vi "Frame Page.vi"(8 "error in (no error)":errorcluster, 11 "Node Ptr":T2 format="%.0x") -> (0 "error out":errorcluster)   [LabVIEW 2019, in "Protection and Counter Addon System Explorer.lvlib"]
uses:
  Protection and Counter Addon System Explorer.lvlib
  <vilib>/NI VeriStand/Custom Device API/Custom Device Item Ref.ctl
  NationalInstruments.VeriStand.SystemStorageUI
  Types/Event Trigger Type.ctl
  <vilib>/NI VeriStand/UI Controls/Single Node Browser/Net Event Data.ctl
  <vilib>/NI VeriStand/UI Controls/Single Node Browser/Net Event.ctl
  Addon Shared/SubVIs/GUID Lookup.vi
  <vilib>/NI VeriStand/Custom Device API/Custom Device API.lvlib
  <vilib>/NI VeriStand/UI Controls/Single Node Browser/NI_VS UI Single Node Browser.lvlib
  Addon Shared/Protection and Counter Addon Shared.lvlib
panel:
  in  "Transmit Trigger":T1
  in  "Trigger":refnum<k24>(container)
  in  "Trigger Settings":cluster{"Section Name":string}={"Section Name"="Transmission Trigger"}
  in  "Trigger":refnum<k24>(container)
  in  "Disable Transmission":bool
  in  "Disable Settings":cluster{"Section Name":string}={"Section Name"="Disable Transmission"}
  in  "Description":string
  out "Frame ID":u32 format="%.0x"
  in  "Custom Device Settings":cluster{"Section Name":string}={"Section Name"="Frame Settings"}
  out "Name":string
  in  "SHDocVw.IWebBrowser2":refnum<k7>(container)
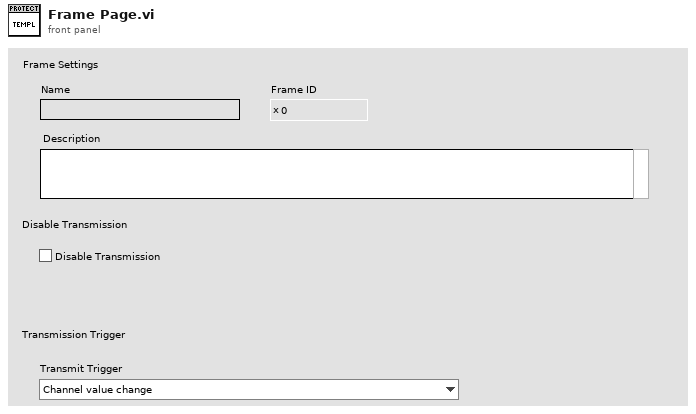
[diagram p1: front panel]
types:
  T1 = typedef "Protection and Counter Addon System Explorer.lvlib/Event Trigger Type.ctl" = enum16{"Channel value change", "Trigger channel (not zero)", "Channel value change or trigger channel (not zero)", "Trigger channel (any value change)", "Channel value change or trigger channel (any value change)"}
  T2 = typedef "Custom Device API.lvlib/Custom Device Item Ref.ctl" = u64
  T3 = cluster{"Trigger":refnum<user-event>, "Transmission":refnum<user-event>}
  T4 = typedef "Protection and Counter Addon System Explorer.lvlib/Frame Settings.ctl" = cluster{"ID":u32, "Disable Transmission":bool, "Disable Transmission Ref":T2, "Transmit Trigger":T1, "Transmit Trigger Ref":T2}
  T5 = typedef "Custom Device API.lvlib/Custom Device Item Info.ctl" = cluster{"Name":string, "Is Channel":bool, "GUID":string, "Is Waveform":bool}
  T6 = typedef "NI_VS UI Single Node Browser.lvlib/Single Node Browser Ref.ctl" = refnum<k24>
  T7 = typedef "NI_VS UI Single Node Browser.lvlib/Callback Type.ctl" = cluster{"Net Callbacks":refnum<k27>[], "Event":refnum<user-event>}
  T8 = typedef "Custom Device API.lvlib/Custom Device Commands.ctl" = enum16{"Default", "Item renamed", "Shutdown", "Dynamic button pressed"}
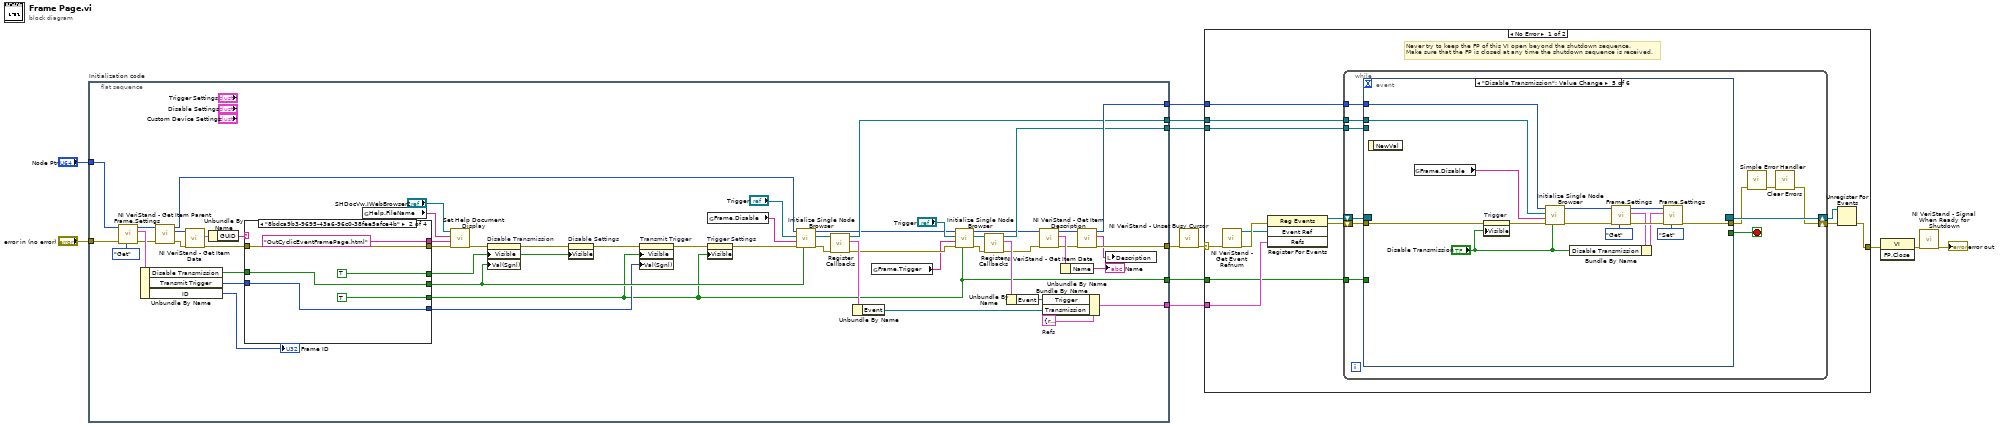
[diagram p0: block diagram]
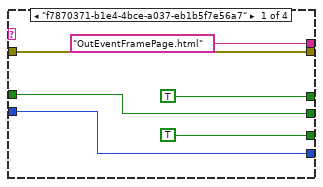
[diagram p2: hidden frame]
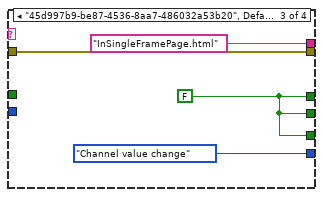
[diagram p3: hidden frame]
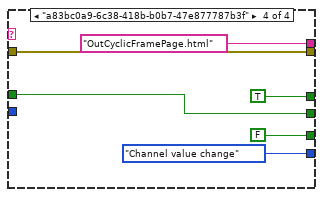
[diagram p4: hidden frame]
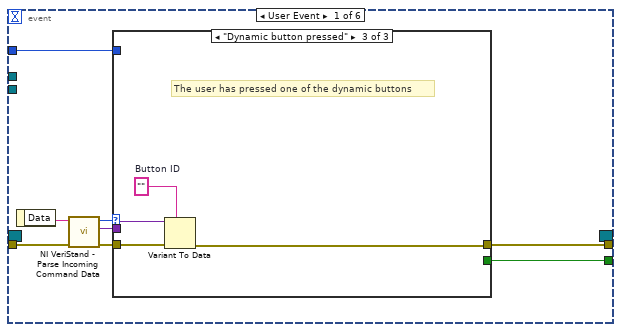
[diagram p5: hidden frame]
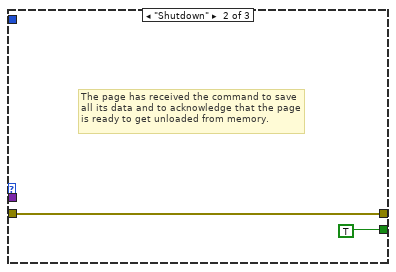
[diagram p7: hidden frame]
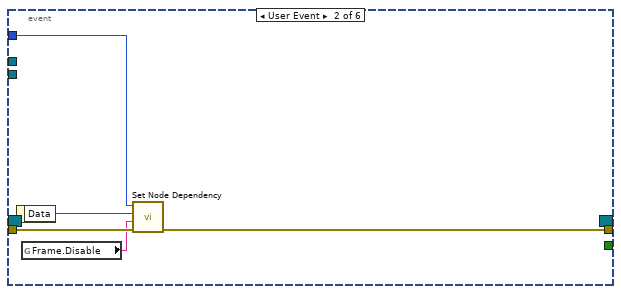
[diagram p8: hidden frame]
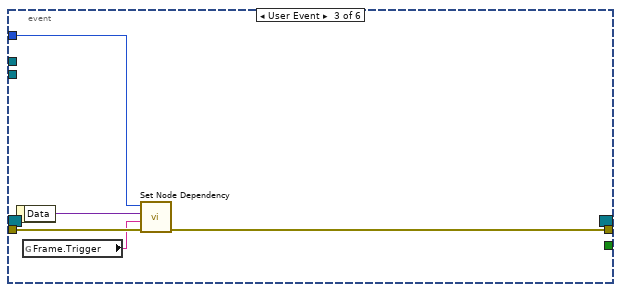
[diagram p9: hidden frame]
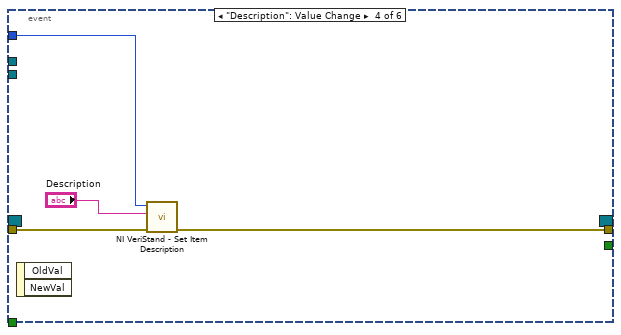
[diagram p10: hidden frame]
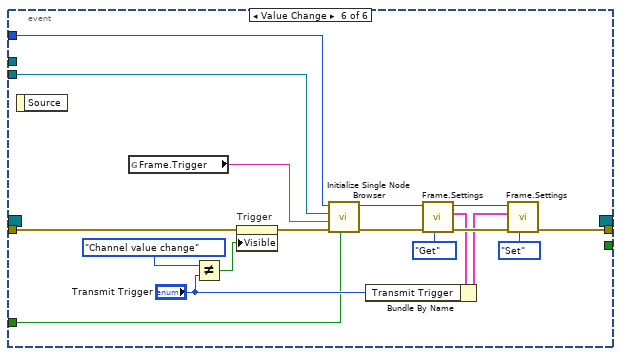
[diagram p11: hidden frame]
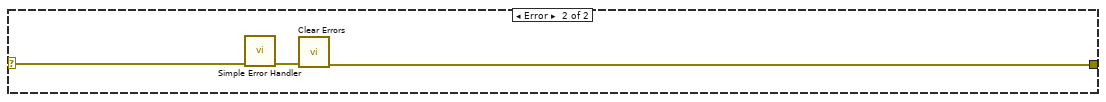
[diagram p12: hidden frame]
diagram:
  n1 = flat-sequence "Initialization code" {
    tunnel: "error in (no error)" -> [w23]
    tunnel: "Node Ptr" -> [w21]
    tunnel: [w62] -> w7
    tunnel: [w60] -> w5
    tunnel: [w44] -> w4
    tunnel: [w46] -> w3
    tunnel: [w36] -> w2
    tunnel: [w16] -> w1
    frame #0 {
      w39 = T3 {"Trigger"=refnum, "Transmission"=refnum}  # Refs
      n2 = call "Frame.Settings.vi"("Action"=enum8{"Get", "Set"}."Get", "error in (no error)"=w23, "Item Ref in"=w21) -> ("error out"=w22:errorcluster, "Frame.Settings"=w27:T4, "Item Ref out"=w20:T2)  [unwired: 6 in]
      n3 = Unbundle By Name(w27) -> ("Disable Transmission"=w19:bool, "Transmit Trigger"=w18:T1, "ID"=→"Frame ID":u32)
      n4 = call <vilib>:"NI VeriStand - Get Item Parent.vi"("error in (no error)"=w22, "Item Ref in"=w20) -> ("error out"=w58:errorcluster, "Parent Ref"=w57:T2, "Item Ref out"=w50:T2)  [unwired: 6 in, 1 out]
      n5 = call <vilib>:"NI VeriStand - Get Item Data.vi"("error in (no error)"=w58, "Item Ref in"=w57) -> ("error out"=w54:errorcluster, "Item Info"=w56:T5)  [unwired: 8 out]
      n6 = Unbundle By Name(w56) -> ("GUID"=w55:string)
      n7 = case shown="\"8bdca9b3-9695-43a6-96c0-38fee5afce4b\"" w55 {
        tunnel: ["OutEventFramePage.html" ("HTML File") "OutCyclicEventFramePage.html" ("HTML File") "InSingleFramePage.html" ("HTML File") "OutCyclicFramePage.html" ("HTML File")] -> w66
        tunnel: w54 -> [w72 w78 w82 w88]
        tunnel: [w72 w78 w82 w88] -> w29
        tunnel: [TRUE TRUE w81 TRUE] -> w47
        tunnel: [w68 w74 w81 w85] -> w31
        tunnel: [TRUE TRUE w81 FALSE] -> w16
        tunnel: [w69 w75 Event_Trigger_Type."Channel value change" ("y") Event_Trigger_Type."Channel value change" ("y")] -> w30
        tunnel: w19 -> [w68 w74 _ w85]
        tunnel: w18 -> [w69 w75 _ _]
        frame "f7870371-b1e4-4bce-a037-eb1b5f7e56a7" {
        }
        frame "8bdca9b3-9695-43a6-96c0-38fee5afce4b" {
        }
        frame "45d997b9-be87-4536-8aa7-486032a53b20", Default {
          w81 = FALSE
        }
        frame "a83bc0a9-6c38-418b-b0b7-47e877787b3f" {
        }
      }
      n8 = global read "GUID Lookup.vi" "Help.FileName"() -> (w13:string)
      n9 = call "Set Help Document Display.vi"("error in (no error)"=w29, "HTML File"=w66, "Main CHM File"=w13, "SHDocVw.IWebBrowser2"="SHDocVw.IWebBrowser2") -> ("error out"=w28:errorcluster)  [unwired: 7 in]
      n10 = property on="Disable Transmission" class="Bool (strict)"(error in=w28, "Visible"=w47, "Val(Sgnl)"=w31) -> (error out=w53:errorcluster)  [unwired: 1 in, 1 out]
      n11 = property on="Disable Settings" class="Clust (strict)"(error in=w53, "Visible"=w47) -> (error out=w33:errorcluster)  [unwired: 1 in, 1 out]
      n12 = property on="Transmit Trigger" class="Enum (strict)"(error in=w33, "Visible"=w16, "Val(Sgnl)"=w30) -> (error out=w32:errorcluster)  [unwired: 1 in, 1 out]
      n13 = property on="Trigger Settings" class="Clust (strict)"(error in=w32, "Visible"=w16) -> (error out=w34:errorcluster)  [unwired: 1 in, 1 out]
      n14 = global read "GUID Lookup.vi" "Frame.Disable"() -> (w15:string)
      n15 = call "Initialize Single Node Browser.vi"("Use Channel?"=w31, "error in (no error)"=w34, "NodeName"=w15, "Browser Ref 2"="Trigger", "Item Ref in"=w50) -> ("error out"=w52:errorcluster, "Browser Ref"=w51:T6, "Item Ref out"=w35:T2)  [unwired: 4 in]
      n16 = call <vilib>:"Register Callbacks.vi"("error in (no error)"=w52, "Single Node Browser"=w51) -> ("error out"=w40:errorcluster, "Callbacks"=w49:T7, "Single Node Browser dup"=w46:T6)  [unwired: 7 in]
      n17 = Unbundle By Name(w49) -> ("Event"=w45:refnum<user-event>)
      n18 = global read "GUID Lookup.vi" "Frame.Trigger"() -> (w14:string)
      n19 = call "Initialize Single Node Browser.vi"("Use Channel?"=w16, "error in (no error)"=w40, "NodeName"=w14, "Browser Ref 2"="Trigger", "Item Ref in"=w35) -> ("error out"=w41:errorcluster, "Browser Ref"=w42:T6, "Item Ref out"=w24:T2)  [unwired: 4 in]
      n20 = call <vilib>:"Register Callbacks.vi"("error in (no error)"=w41, "Single Node Browser"=w42) -> ("error out"=w25:errorcluster, "Callbacks"=w43:T7, "Single Node Browser dup"=w36:T6)  [unwired: 7 in]
      n21 = Unbundle By Name(w43) -> ("Event"=w38:refnum<user-event>)
      n22 = call <vilib>:"NI VeriStand - Get Item Data.vi"("error in (no error)"=w25, "Item Ref in"=w24) -> ("error out"=w63:errorcluster, "Item Info"=w65:T5, "Item Ref out"=w61:T2)  [unwired: 7 out]
      n23 = Bundle By Name(cluster=w39, "Trigger"=w38, "Transmission"=w45) -> (w44:T3)
      n24 = Unbundle By Name(w65) -> ("Name"=→"Name":string)
      n25 = call <vilib>:"NI VeriStand - Get Item Description.vi"("error in (no error)"=w63, "Item Ref in"=w61) -> ("error out"=w62:errorcluster, "Description"=w59:string, "Item Ref out"=w60:T2)  [unwired: 7 out]
      n26 = local write "Description"(w59) -> ()
    }
  }
  n27 = call <vilib>:"NI VeriStand - Unset Busy Cursor.vi"("error in (no error)"=w7) -> ("error out"=w9:errorcluster)  [unwired: 10 out]
  n28 = case shown="No Error" w9 {
    selector: w9 -> [w94 w178]
    tunnel: [w99 w176] -> w12
    tunnel: w5 -> [w95 _]
    tunnel: w4 -> [w93 _]
    tunnel: w3 -> [w92 _]
    tunnel: w2 -> [w91 _]
    tunnel: w1 -> [w90 _]
    frame No Error {
      # "Never try to keep the FP of this VI open beyond the shutdown sequence.\nMake sure that the FP is closed at any time the shutdown sequence is received."
      n29 = call <vilib>:"NI VeriStand - Get Event Refnum.vi"("error in (no error)"=w94) -> ("error out"=w102:errorcluster, "Event Ref"=w98:refnum<user-event>)  [unwired: 9 out]
      n30 = register-events(error in=w102, w98, w93) -> (reference out=w96:refnum<event-registration>, error out=w97:errorcluster)  [unwired: 1 in]
      n31 = while {
        tunnel: w95 -> [w109]
        shift-right: [w106] -> w100
        shift-left: w97 -> [w112]
        shift-right: [w113] -> w101
        shift-left: w96 -> [w111]
        tunnel: w92 -> [w105]
        tunnel: w91 -> [w104]
        tunnel: w90 -> [w103]
        stop <- w110 stop-if-true
        n32 = event shown="[4] \"Disable Transmission\": Value Change" {
          selector: w111 -> [_ _ _ _ _ _]
          dyn-events: [_ _ _ _ _ _] -> w113
          timeout: _ -> [_ _ _ _ _ _]
          tunnel: w112 -> [w121 w131 w136 w142 w157 w175]
          tunnel: [w117 _ _ _ _ _] -> w110
          tunnel: [w116 w130 w135 w141 w148 w162] -> w108
          tunnel: w109 -> [w115 w132 w137 w140 w155 w174]
          tunnel: w105 -> [_ _ _ _ w156 _]
          tunnel: w104 -> [_ _ _ _ _ w170]
          tunnel: w103 -> [_ _ _ _ _ w160]
          event User Event {
            n33 = event-data() -> ("Data"=w120:string)  [unwired: 1 out]
            n34 = call <vilib>:"NI VeriStand - Parse Incoming Command Data.vi"("error in (no error)"=w121, "Incoming data"=w120) -> ("error out"=w119:errorcluster, "Outgoing data"=w114:variant, "Action"=w118:T8)  [unwired: 7 out]
            n35 = case shown="\"Dynamic button pressed\"" w118 {
              tunnel: w119 -> [w122 w123 w128]
              tunnel: [_ TRUE _] -> w117
              tunnel: [w122 w123 w125] -> w116
              tunnel: w115 -> [_ _ _]
              tunnel: w114 -> [_ _ w127]
              frame "Default", Default {
              }
              frame "Shutdown" {
                # "The page has received the command to save all its data and to acknowledge that the page is ready to get unloaded from memory."
              }
              frame "Dynamic button pressed" {
                w126 = ""  # Button ID
                # "The user has pressed one of the dynamic buttons"
                n36 = Variant To Data(error in=w128, type=w126, Variant=w127) -> (error out=w125:errorcluster)  [unwired: 1 out]
              }
            }
          }
          event User Event {
            n37 = event-data() -> ("Data"=w133:variant)  [unwired: 1 out]
            n38 = global read "GUID Lookup.vi" "Frame.Disable"() -> (w129:string)
            n39 = call "Set Node Dependency.vi"("error in (no error)"=w131, "NodeName"=w129, "Data"=w133, "Item Ref in"=w132) -> ("error out"=w130:errorcluster)  [unwired: 6 in, 1 out]
          }
          event User Event {
            n40 = event-data() -> ("Data"=w138:variant)  [unwired: 1 out]
            n41 = global read "GUID Lookup.vi" "Frame.Trigger"() -> (w134:string)
            n42 = call "Set Node Dependency.vi"("error in (no error)"=w136, "NodeName"=w134, "Data"=w138, "Item Ref in"=w137) -> ("error out"=w135:errorcluster)  [unwired: 6 in, 1 out]
          }
          event "Description": Value Change {
            n43 = event-data() -> ()  [unwired: 3 out]
            n44 = call <vilib>:"NI VeriStand - Set Item Description.vi"("error in (no error)"=w142, "Description"="Description", "Item Ref in"=w140) -> ("error out"=w141:errorcluster)  [unwired: 8 out]
          }
          event "Disable Transmission": Value Change {
            n45 = event-data() -> ()  [unwired: 2 out]
            n46 = global read "GUID Lookup.vi" "Frame.Disable"() -> (w143:string)
            n47 = property on="Trigger" class="AXCont"(error in=w157, "Visible"="Disable Transmission") -> (error out=w154:errorcluster)  [unwired: 1 in, 1 out]
            n48 = call "Initialize Single Node Browser.vi"("Use Channel?"="Disable Transmission", "error in (no error)"=w154, "NodeName"=w143, "Browser Ref 2"=w156, "Item Ref in"=w155) -> ("error out"=w151:errorcluster, "Item Ref out"=w152:T2)  [unwired: 4 in, 1 out]
            n49 = call "Frame.Settings.vi"("Action"=enum8{"Get", "Set"}."Get", "error in (no error)"=w151, "Item Ref in"=w152) -> ("error out"=w149:errorcluster, "Frame.Settings"=w146:T4, "Item Ref out"=w147:T2)  [unwired: 6 in]
            n50 = Bundle By Name(cluster=w146, "Disable Transmission"="Disable Transmission") -> (w144:T4)
            n51 = call "Frame.Settings.vi"("Action"=enum8{"Get", "Set"}."Set", "error in (no error)"=w149, "Frame.Settings"=w144, "Item Ref in"=w147) -> ("error out"=w148:errorcluster)  [unwired: 5 in, 2 out]
          }
          event Value Change {
            n52 = event-data() -> ()  [unwired: 2 out]
            n53 = global read "GUID Lookup.vi" "Frame.Trigger"() -> (w158:string)
            n54 = Not Equal?(x=Event_Trigger_Type."Channel value change" ("y"), y="Transmit Trigger") -> (x != y?=w171:bool)
            n55 = property on="Trigger" class="AXCont"(error in=w175, "Visible"=w171) -> (error out=w173:errorcluster)  [unwired: 1 in, 1 out]
            n56 = call "Initialize Single Node Browser.vi"("Use Channel?"=w160, "error in (no error)"=w173, "NodeName"=w158, "Browser Ref 2"=w170, "Item Ref in"=w174) -> ("error out"=w163:errorcluster, "Item Ref out"=w161:T2)  [unwired: 4 in, 1 out]
            n57 = call "Frame.Settings.vi"("Action"=enum8{"Get", "Set"}."Get", "error in (no error)"=w163, "Item Ref in"=w161) -> ("error out"=w167:errorcluster, "Frame.Settings"=w165:T4, "Item Ref out"=w166:T2)  [unwired: 6 in]
            n58 = Bundle By Name(cluster=w165, "Transmit Trigger"="Transmit Trigger") -> (w159:T4)
            n59 = call "Frame.Settings.vi"("Action"=enum8{"Get", "Set"}."Set", "error in (no error)"=w167, "Frame.Settings"=w159, "Item Ref in"=w166) -> ("error out"=w162:errorcluster)  [unwired: 5 in, 2 out]
          }
        }
        n60 = call <vilib>:"Simple Error Handler.vi"("error in (no error)"=w108) -> ("error out"=w107:errorcluster)  [unwired: 1 in, 7 out]
        n61 = call <vilib>:"Clear Errors.vi"("error in (no error)"=w107) -> ("error out"=w106:errorcluster)  [unwired: 1 in, 5 out]
      }
      n62 = Unregister For Events(event registration refnum=w101, error in=w100) -> (error out=w99:errorcluster)
    }
    frame Error {
      n63 = call <vilib>:"Simple Error Handler.vi"("error in (no error)"=w178) -> ("error out"=w177:errorcluster)  [unwired: 1 in, 7 out]
      n64 = call <vilib>:"Clear Errors.vi"("error in (no error)"=w177) -> ("error out"=w176:errorcluster)  [unwired: 1 in, 5 out]
    }
  }
  n65 = invoke class="VI" method="FP.Close"(error in=w12) -> (error out=w11:errorcluster)  [unwired: 2 in, 2 out]
  n66 = call <vilib>:"NI VeriStand - Signal When Ready for Shutdown.vi"("error in (no error)"=w11) -> ("error out"=→"error out":errorcluster)  [unwired: 10 out]
